vi "Configure Average.vi"(7 "Average on":bool, 8 "error in (no error)":errorcluster, 10 "Average Count":i32, 11 "RS Z2X in":refnum<class "RS Z2X.lvclass">) -> (0 "error out":errorcluster, 3 "RS Z2X out":refnum<class "RS Z2X.lvclass">)   [LabVIEW 2020, in "RS Z2X.lvclass"]
uses:
  RS Z2X.lvclass
  C:/Sandbox/Git_Sandbox/WiSpry Test Framework source code (LV20)/WiSpry Test Framework/Instruments/Instrument.lvclass
  C:/Sandbox/Git_Sandbox/WiSpry Test Framework source code (LV20)/WiSpry Test Framework/Instruments/Power Meter/Power Meter.lvclass
  Instrument.lvclass/Instrument.ctl
  Power Meter.lvclass/Power Meter.ctl
  Instrument.lvclass
  Power Meter.lvclass
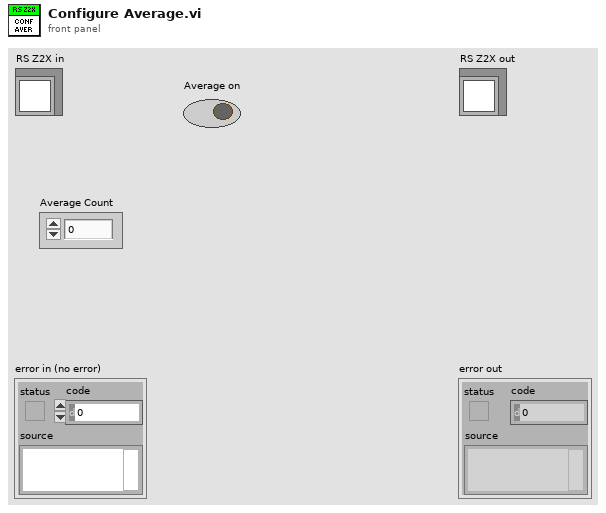
[diagram p1: front panel]
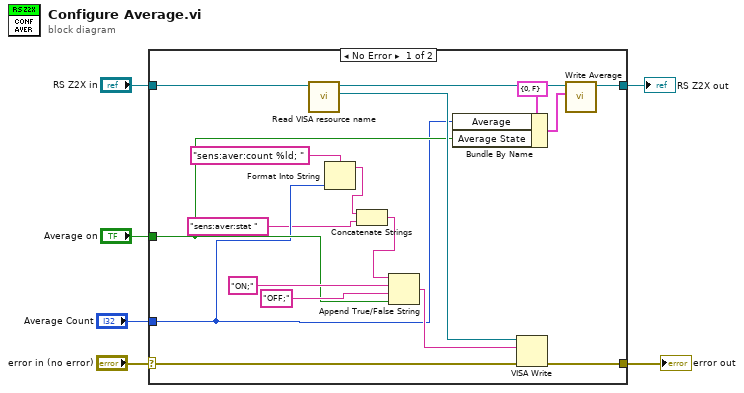
[diagram p0: block diagram]
diagram:
  n1 = case shown="No Error" "error in (no error)" {
    selector: "error in (no error)" -> [w21 w25]
    tunnel: "RS Z2X in" -> [w23 w24]
    tunnel: [w20 w25] -> w2
    tunnel: "Average on" -> [w13 _]
    tunnel: "Average Count" -> [w10 _]
    tunnel: [w18 w24] -> w1
    frame No Error {
      n2 = call "Read VISA resource name.vi"("Instrument in"=w23) -> ("VISA resource name"=w22:refnum<visa-resource-name>, "Instrument out"=w19:refnum<class "RS Z2X.lvclass">)  [unwired: 9 in]
      n3 = Format Into String(format string="sens:aver:count %ld; " ("string (\"\")"), w10) -> (resulting string=w9:string)  [unwired: 2 in, 1 out]
      n4 = Concatenate Strings(w9, "sens:aver:stat " ("string (\"\")")) -> (w7:string)
      n5 = Append True/False String(1:w13, 2:"OFF;" ("false string"), 3:"ON;" ("true string"), 4:w7) -> (0:w11:string)
      n6 = Bundle By Name(cluster=cluster{"Average":i32, "Average State":bool} {"Average"=0, "Average State"=FALSE} ("Average"), "Average"=w10, "Average State"=w13) -> (w16:cluster{"Average":i32, "Average State":bool})
      n7 = VISA Write(VISA resource name=w22, write buffer=w11, error in (no error)=w21) -> (error out=w20:errorcluster)  [unwired: 2 out]
      n8 = call "Write Average.vi"("Average"=w16, "Power Meter in"=w19) -> ("Power Meter out"=w18:refnum<class "RS Z2X.lvclass">)  [unwired: 9 in]
    }
    frame Error {
    }
  }
  "error out" <- w2
  "RS Z2X out" <- w1
